vi "JuPyter_Client_Init.vi"(8 "error in (no error)":errorcluster, 11 "object in":refnum<class "JuPyter_Client.lvclass">) -> (0 "error out":errorcluster, 3 "object out":refnum<class "JuPyter_Client.lvclass">)   [LabVIEW 2018, in "JuPyter_Client.lvclass"]
uses:
  JuPyter_Client.lvclass
  JuPyter_Client.lvclass/JuPyter_Client.ctl
  <vilib>/addons/zeromq/zmq_context.lvclass
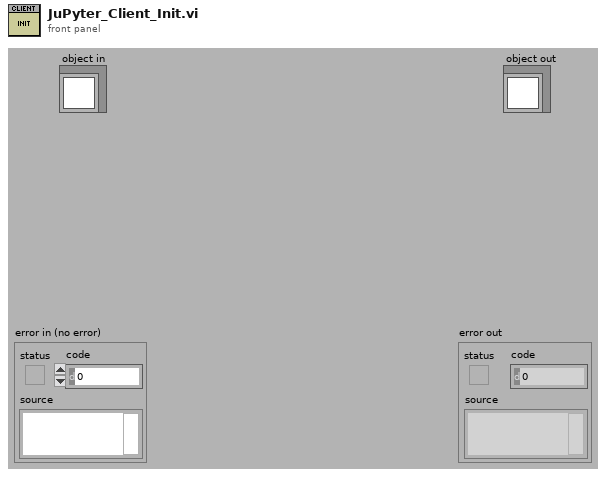
[diagram p1: front panel]
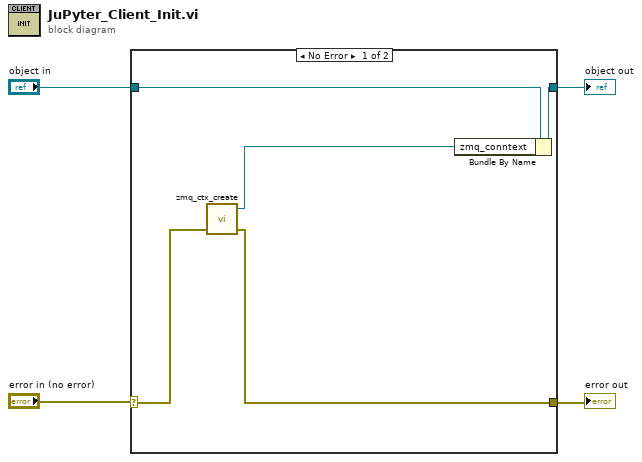
[diagram p0: block diagram]
diagram:
  n1 = case shown="No Error" "error in (no error)" {
    selector: "error in (no error)" -> [w6 w10]
    tunnel: "object in" -> [w9 w11]
    tunnel: [w8 w11] -> w3
    tunnel: [w5 w10] -> w1
    frame No Error {
      n2 = call <vilib>:"zmq_ctx_create.vi"("error in"=w6) -> ("error out"=w5:errorcluster, "context out"=w7:refnum<class "zmq_context.lvclass">)  [unwired: 3 in]
      n3 = Bundle By Name(cluster=w9, "zmq_conntext"=w7) -> (w8:refnum<class "JuPyter_Client.lvclass">)
    }
    frame Error {
    }
  }
  "object out" <- w3
  "error out" <- w1
